vi "prepare image for 2nd mom analysis.vi"(8 "error in (no error)":errorcluster, 11 "FakeCamera in":refnum<class "Point Grey Camera.lvclass">) -> (0 "error out":errorcluster, 2 "BG sub image":T1(plugin-control), 3 "thresholded for 2nd mom":T1, 5 "FakeCamera out":refnum<class "Point Grey Camera.lvclass">)   [LabVIEW 2020, in "Point Grey Camera.lvclass"]
uses:
  Point Grey Camera.lvclass
  IMAQ Image.ctl
  Point Grey Camera.lvclass/Point Grey Camera.ctl
  NI_Vision_Development_Module.lvlib
panel:
  out "Optional Rectangle":i32[](array[numeric])=[192, 108, 374, 256]
  in  "Median rank":i32
  out "thresh for 2nd mom out":T1
  out "BG sub image 45":T1(plugin-control)
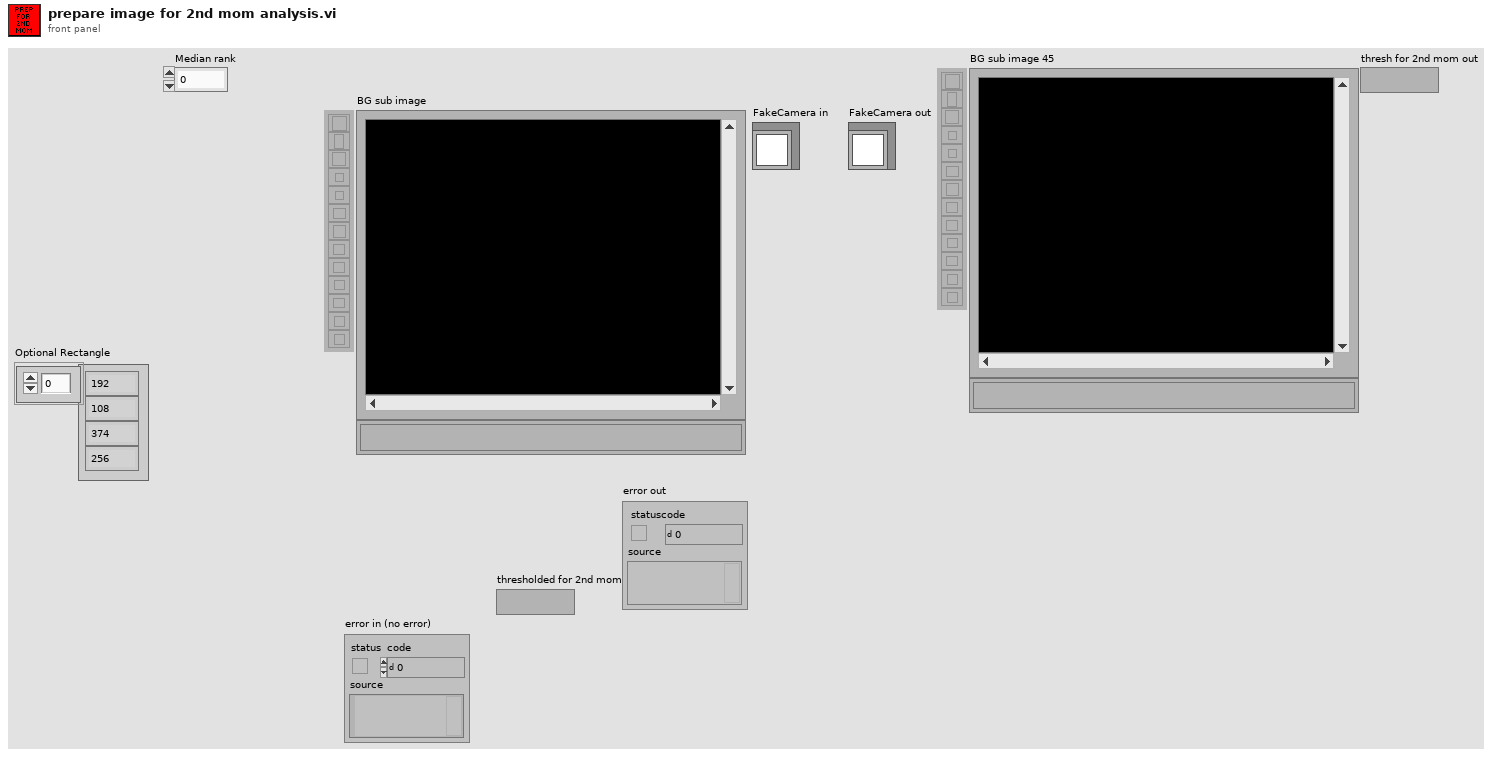
[diagram p1: front panel]
types:
  T1 = typedef "IMAQ Image.ctl" = refnum<image>
  T2 = typedef "Image Type" = u32
  T3 = typedef "OnOffTypeDef.ctl" = enum16{"off", "on"}
  T4 = cluster{"X Size":i32, "Y Size":i32, "Order #":i32}
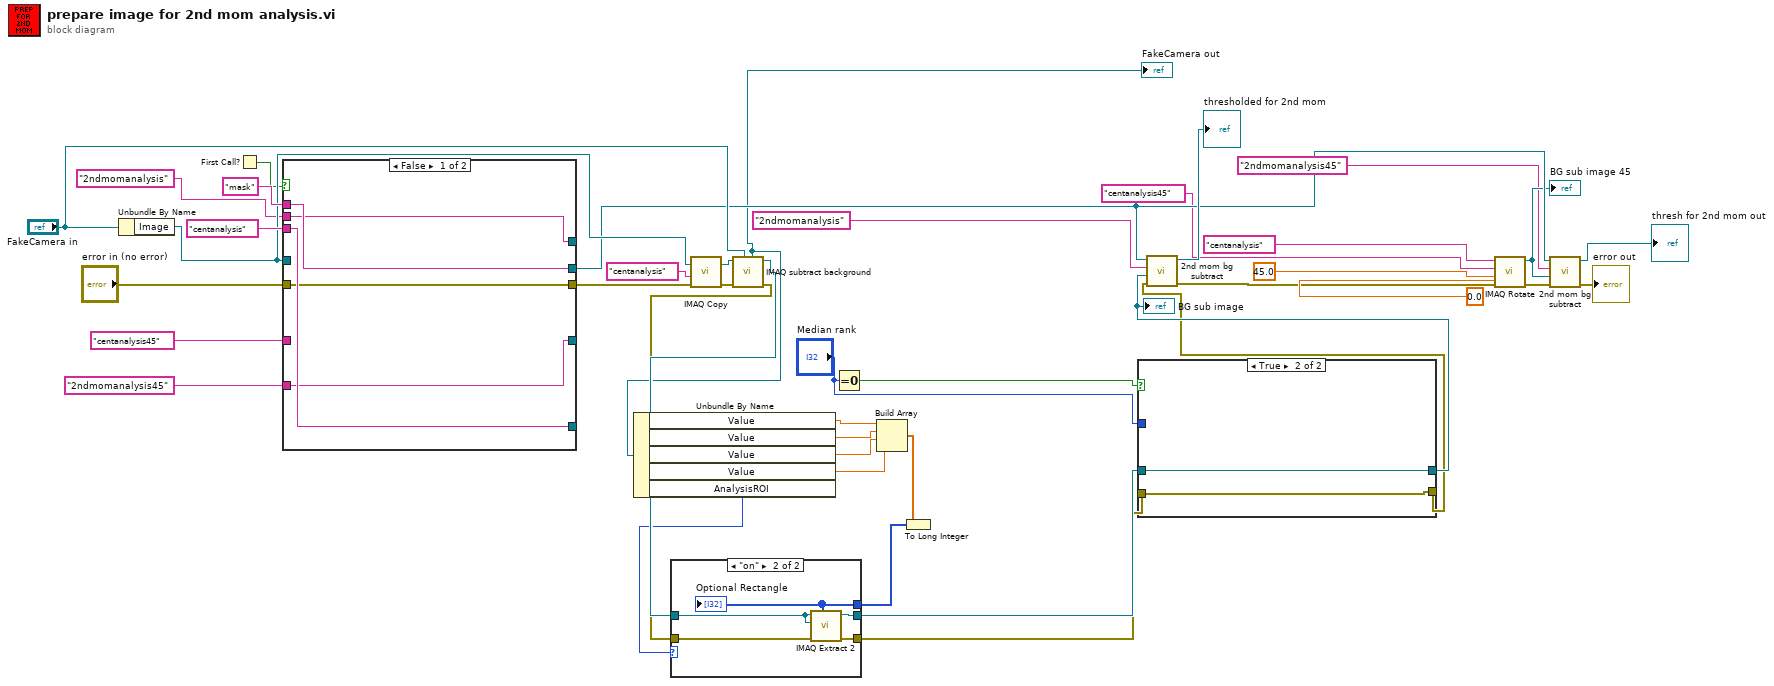
[diagram p0: block diagram]
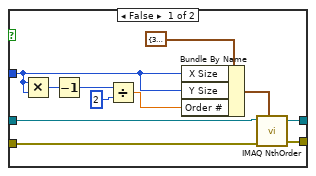
[diagram p3: hidden frame]
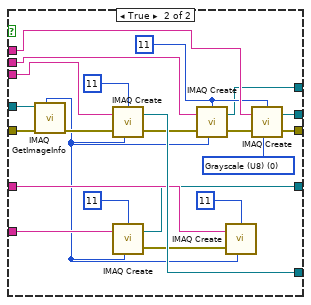
[diagram p4: hidden frame]
diagram:
  n1 = Unbundle By Name("FakeCamera in") -> ("Image"=w38:T1)
  n2 = First Call?() -> (First Call?: T/F=w35:bool)
  n3 = case shown="False" w35 {
    tunnel: [w47 w69] -> w27
    tunnel: "mask" ("Image Name") -> [w47 w67]
    tunnel: "centanalysis" ("Image Name") -> [w45 w63]
    tunnel: "error in (no error)" -> [w44 w59]
    tunnel: w38 -> [_ w61]
    tunnel: "2ndmomanalysis" ("Image Name") -> [w46 w60]
    tunnel: [w44 w58] -> w32
    tunnel: [w46 w57] -> _
    tunnel: [w45 w56] -> _
    tunnel: "2ndmomanalysis45" ("Image Name") -> [w43 w53]
    tunnel: "centanalysis45" ("Image Name") -> [_ w51]
    tunnel: [w43 w49] -> _
    frame False {
    }
    frame True {
      w68 = T2 0 items=["Grayscale (U8)", "Grayscale (I16)", "Grayscale (SGL)", "Complex (CSG)", "RGB (U32)", "HSL (U32)", "RGB (U64)", "Grayscale (U16)"] ("Image Type")
      w62 = 11 ("Border Size")
      n4 = call "IMAQ GetImageInfo"("error in (no error)"=w59, "Image"=w61) -> ("error out"=w65:errorcluster, "Image Type"=w48:T2)  [unwired: 2 in, 6 out]
      n5 = call "IMAQ Create"("Border Size"=11, "Image Name"=w63, "Image Type"=w48, "error in (no error)"=w65) -> ("New Image"=w56:T1, "error out"=w55:errorcluster)  [unwired: 1 in]
      n6 = call "IMAQ Create"("Border Size"=11, "Image Name"=w53, "Image Type"=w48) -> ("New Image"=w49:T1, "error out"=w50:errorcluster)  [unwired: 2 in]
      n7 = call "IMAQ Create"("Border Size"=w62, "Image Name"=w60, "Image Type"=w48, "error in (no error)"=w55) -> ("New Image"=w57:T1, "error out"=w66:errorcluster)  [unwired: 1 in]
      n8 = call "IMAQ Create"("Border Size"=11, "Image Name"=w51, "Image Type"=w48, "error in (no error)"=w50) -> ()  [unwired: 1 in, 2 out]
      n9 = call "IMAQ Create"("Border Size"=w62, "Image Name"=w67, "Image Type"=w68, "error in (no error)"=w66) -> ("New Image"=w69:T1, "error out"=w58:errorcluster)  [unwired: 1 in]
    }
  }
  n10 = call "IMAQ Copy"("error in (no error)"=w32, "Image Dst"="centanalysis" ("Image Name"), "Image Src"=w38) -> ("error out"=w34:errorcluster, "Image Dst Out"=w33:T1)  [unwired: 3 in]
  n11 = call "IMAQ subtract background.vi"("FakeCamera in"="FakeCamera in", "error in (no error)"=w34, "Image in"=w33) -> ("error out"=w11:errorcluster, "Refnum out"=w13:T1, "FakeCamera out"=w8:refnum<class "Point Grey Camera.lvclass">)  [unwired: 3 in, 3 out]
  "FakeCamera out" <- w8
  n12 = Unbundle By Name(w8) -> ("Value"=w7:dbl, "Value"=w6:dbl, "Value"=w5:dbl, "Value"=w4:dbl, "AnalysisROI"=w1:T3)
  n13 = Equal To 0?(x="Median rank") -> (x = 0?=w14:bool)
  n14 = Build Array(w7, w6, w5, w4) -> (w3:dbl[])
  n15 = To Long Integer(number=w3) -> (32bit integer=w2:i32[])
  n16 = case shown="\"on\"" w1 {
    tunnel: w13 -> [w71 w76]
    tunnel: [w71 w75] -> w12
    tunnel: w11 -> [w70 w74]
    tunnel: [w70 w73] -> w10
    tunnel: w2 -> [_ w72]
    frame "off", Default {
    }
    frame "on" {
      n17 = call "IMAQ Extract 2"("Optional Rectangle"=w72, "error in (no error)"=w74, "Image Dst"=w76, "Image Src"=w76) -> ("error out"=w73:errorcluster, "Image Dst Out"=w75:T1)  [unwired: 6 in]
      "Optional Rectangle" <- w72
    }
  }
  n18 = case shown="True" w14 {
    tunnel: w12 -> [w87 w89]
    tunnel: [w81 w89] -> w16
    tunnel: "Median rank" -> [w79 _]
    tunnel: w10 -> [w78 w88]
    tunnel: [w77 w88] -> w9
    frame False {
      n19 = Multiply(x=w79, y=w79) -> (x*y=w85:i32)
      n20 = Decrement(x=w85) -> (x-1=w84:i32)
      n21 = Divide(x=w84, y=2) -> (x/y=w82:dbl)
      n22 = Bundle By Name(cluster=T4 {"X Size"=3, "Y Size"=3, "Order #"=4} ("Size & Order #"), "X Size"=w79, "Y Size"=w79, "Order #"=w82) -> (w80:T4)
      n23 = call "IMAQ NthOrder"("Image Src"=w87, "Size & Order #"=w80, "error in (no error)"=w78) -> ("Image Dst Out"=w81:T1, "error out"=w77:errorcluster)  [unwired: 4 in]
    }
    frame True {
    }
  }
  "BG sub image" <- w16
  n24 = call "2nd mom bg subtract.vi"("error in (no error)"=w9, "BG sub in"=w16, "2ndmom"="2ndmomanalysis" ("Image Name"), "mask"=w27) -> ("error out"=w24:errorcluster, "thresh for 2nd mom out"=→"thresholded for 2nd mom":T1)  [unwired: 6 in]
  n25 = call "IMAQ Rotate"("Replace Value"=sgl 0.0, "error in (no error)"=w24, "Angle (degrees)"=sgl 45.0, "Image Dst"="centanalysis45" ("Image Name"), "Image Src"="centanalysis" ("Image Name")) -> ("error out"=w23:errorcluster, "Image Dst Out"=w26:T1)  [unwired: 5 in]
  "BG sub image 45" <- w26
  n26 = call "2nd mom bg subtract.vi"("error in (no error)"=w23, "BG sub in"=w26, "2ndmom"="2ndmomanalysis45" ("Image Name"), "mask"=w27) -> ("error out"=→"error out":errorcluster, "thresh for 2nd mom out"=→"thresh for 2nd mom out":T1)  [unwired: 6 in]
